vi "DHE_Roi2Center.vi"(10 "roi":string) -> (0 "ybox":i32, 1 "xbox":i32, 2 "yc":i32, 3 "xc":i32)   [LabVIEW 2016]
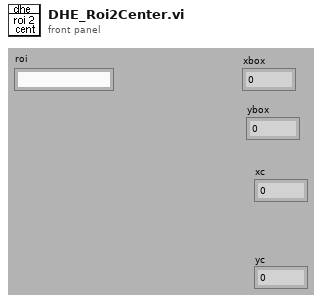
[diagram p1: front panel]
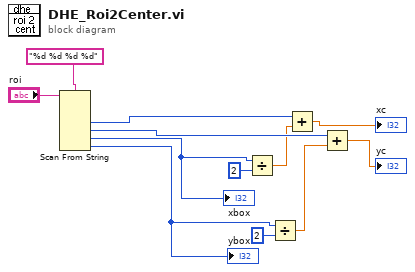
[diagram p0: block diagram]
diagram:
  n1 = Scan From String(format string="%d %d %d %d", input string="roi") -> (output 1=w10:i32, output 2=w9:i32, output 3=w7:i32, output 4=w4:i32)  [unwired: 2 in, 7 out]
  "xbox" <- w7
  "ybox" <- w4
  n2 = Divide(x=w7, y=2) -> (x/y=w6:dbl)
  n3 = Divide(x=w4, y=2) -> (x/y=w3:dbl)
  n4 = Add(x=w10, y=w6) -> (x+y=→"xc":dbl)
  n5 = Add(x=w9, y=w3) -> (x+y=→"yc":dbl)
